vi "Menu Actions.vi"(8 "error in (no error)":errorcluster, 10 "Tag":string, 11 "Self Enqueuer":refnum<class "Message Enqueuer.lvclass">) -> (0 "error out":errorcluster)   [LabVIEW 2016, in "Assert API Components.lvlib" / "Assert Display.lvlib" / "Service Config Display.lvlib" / "Service Config Display.lvclass"]
doc: "Actions a right click menu selection"
uses:
  Service Config Display.lvclass
  <vilib>/ActorFramework/Message Enqueuer/Message Enqueuer.lvclass
  Service Config Display Messages/Add New Service Msg/Add New Service Msg.lvclass/Add New Service Msg.ctl
  <vilib>/ActorFramework/Message Enqueuer/Message Enqueuer.lvclass/Message Enqueuer.ctl
  Service Config Display Messages/Remove Named Service Msg/Remove Named Service Msg.lvclass/Remove Named Service Msg.ctl
  <vilib>/ActorFramework/Message Enqueuer/Enqueue.vi
  Service Config Display Messages/Add New Service Msg/Add New Service Msg.lvclass
  C:/Program Files (x86)/National Instruments/LabVIEW 2016/vi.lib/ActorFramework/Message/Message.lvclass
  Service Config Display Messages/Remove Named Service Msg/Remove Named Service Msg.lvclass
  <vilib>/ActorFramework/Message Priority Queue/Priority Enqueue.vi
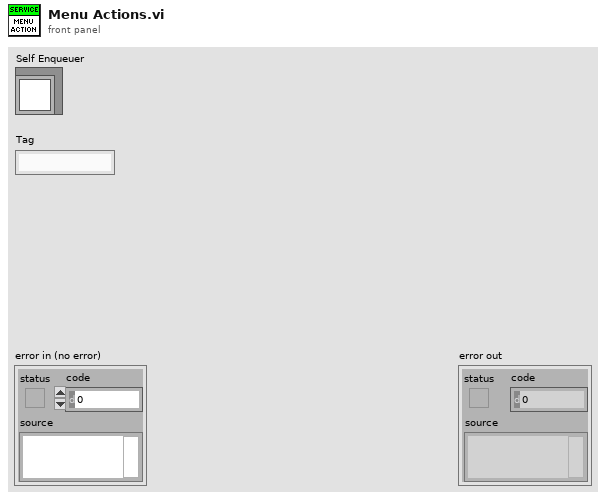
[diagram p1: front panel]
types:
  T1 = typedef "Assert API Components.lvlib/Assert Display.lvlib/Service Details.ctl" = cluster{"Name":string, "IP Address":string}
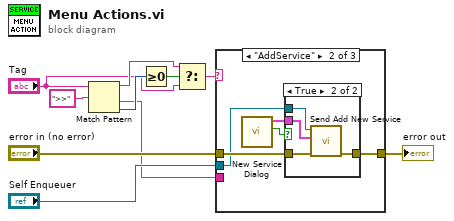
[diagram p0: block diagram]
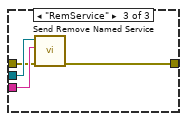
[diagram p4: hidden frame]
diagram:
  n1 = Match Pattern(string="Tag", regular expression=">>") -> (before substring=w4:string, after substring=w1:string, offset past match=w6:i32)  [unwired: 1 in, 1 out]
  n2 = Greater Or Equal To 0?(x=w6) -> (x >= 0?=w5:bool)
  n3 = Select(t=w4, s=w5, f="Tag") -> (s? t:f=w2:string)
  n4 = case shown="\"AddService\"" w2 {
    tunnel: "Self Enqueuer" -> [_ w14 w25]
    tunnel: "error in (no error)" -> [w11 w16 w23]
    tunnel: [w11 w15 w22] -> w8
    tunnel: w1 -> [_ _ w24]
    frame Default {
    }
    frame "AddService" {
      n5 = call "New Service Dialog.vi"() -> ("Create New"=w12:bool, "Service Details"=w13:T1)  [unwired: 10 in]
      n6 = case shown="True" w12 {
        tunnel: w16 -> [w17 w21]
        tunnel: [w17 w20] -> w15
        tunnel: w14 -> [_ w19]
        tunnel: w13 -> [_ w18]
        frame False {
        }
        frame True {
          n7 = call "Send Add New Service.vi"("error in (no error)"=w21, "Service Details"=w18, "Message Enqueuer"=w19) -> ("error out"=w20:errorcluster)  [unwired: 7 in, 1 out]
        }
      }
    }
    frame "RemService" {
      n8 = call "Send Remove Named Service.vi"("error in (no error)"=w23, "Service Name"=w24, "Message Enqueuer"=w25) -> ("error out"=w22:errorcluster)  [unwired: 7 in, 1 out]
    }
  }
  "error out" <- w8
